vi "Temperature Controller.vi"(1 "Action":T7=enum."Identify", 2 "Parameters":variant) -> (6 "Output":variant, 7 "Stop":bool)   [LabVIEW 2024]
doc: "This VI reads a single reading from a Keithley 2001 multimeter. The stop boolean is always false. If no reading is obtained a single zero is returned.\nScott Hannahs, NHMFL-FSU, Nov 1993"
uses:
  Sub Controls/Instrument Actions.ctl
  Sub Controls/Instrument Match.ctl
  Sub Controls/Public.ctl
  Sub Controls/Factory Reset.ctl
  Sub Controls/Scan Output.ctl
  Sub Controls/Instrument IDN.ctl
  Sub Controls/User Event Command.ctl
  <vilib>/Utility/error.llb/Trim Whitespace One-Sided.vi
panel:
  in  "Factory Reset":T1
  in  "CryoCon 62 Channel":enum16{"A", "B"}(ring) caption="Channel"
  in  "LakeShore 372 Channel":T2(ring) caption="Channel"
  out "Instrument Name":string
  in  "LakeShore 370 Channel":T3(ring) caption="Channel"
  in  "LakeShore 340 Channel":enum16{"A", "B", "C", "D"}(ring) caption="Channel"
  in  "Measurement Type":T4(radio)
  out "Title":string
  in  "Public":T5
  in  "Address":u16(ring) items=["GPIB 0 - Address 8", "GPIB 0 - Address 9", "GPIB 0 - Address 11", "GPIB 0 - Address 12", "GPIB 0 - Address 13"]
  out "Model":string
  in  "Instruments":T6[](array[typedef])=[{"Model"="MODEL370", "Manufacturer"="LSCI", "Term Character"="", "Wait Time (mS)"=0, "Wait for SRQ"=FALSE, "Type"="Temperature Controller"}, {"Model"="MODEL340", "Manufacturer"="LSCI", "Term Character"="", "Wait Time (mS)"=0, "Wait for SRQ"=FALSE, "Type"="Temperature Controller"}, {"Model"="MODEL336", "Manufacturer"="LSCI", "Term Character"="", "Wait Time (mS)"=0, "Wait for SRQ"=FALSE, "Type"="Temperature Controller"}, {"Model"="Model 62", "Manufacturer"="Cryocon", "Term Character"="", "Wait Time (mS)"=0, "Wait for SRQ"=FALSE, "Type"="Temperature Controller"}, {"Model"="MODEL372", "Manufacturer"="LSCI", "Term Character"="", "Wait Time (mS)"=0, "Wait for SRQ"=FALSE, "Type"="Temperature Controller"}, {"Model"="24C", "Manufacturer"="Cryo-con", "Term Character"="", "Wait Time (mS)"=0, "Wait for SRQ"=FALSE, "Type"="Temperature Controller"}, {"Model"="Model", "Manufacturer"="Cryocon", "Term Character"="", "Wait Time (mS)"=0, "Wait for SRQ"=FALSE, "Type"="Temperature Controller"}, {"Model"="MODEL331S", "Manufacturer"="LSCI", "Term Character"="", "Wait Time (mS)"=0, "Wait for SRQ"=FALSE, "Type"="Temperature Controller"}]
  out "Measurement":dbl[](array[numeric]) format="%^_7e"
  in  "VISA resource name":refnum<visa-resource-name>
  # "Term Char"
  # "Wait Time (mS)"
  # "Wait for SRQ?"
  # "Type"
  # "Manufacturer"
  # "Model"
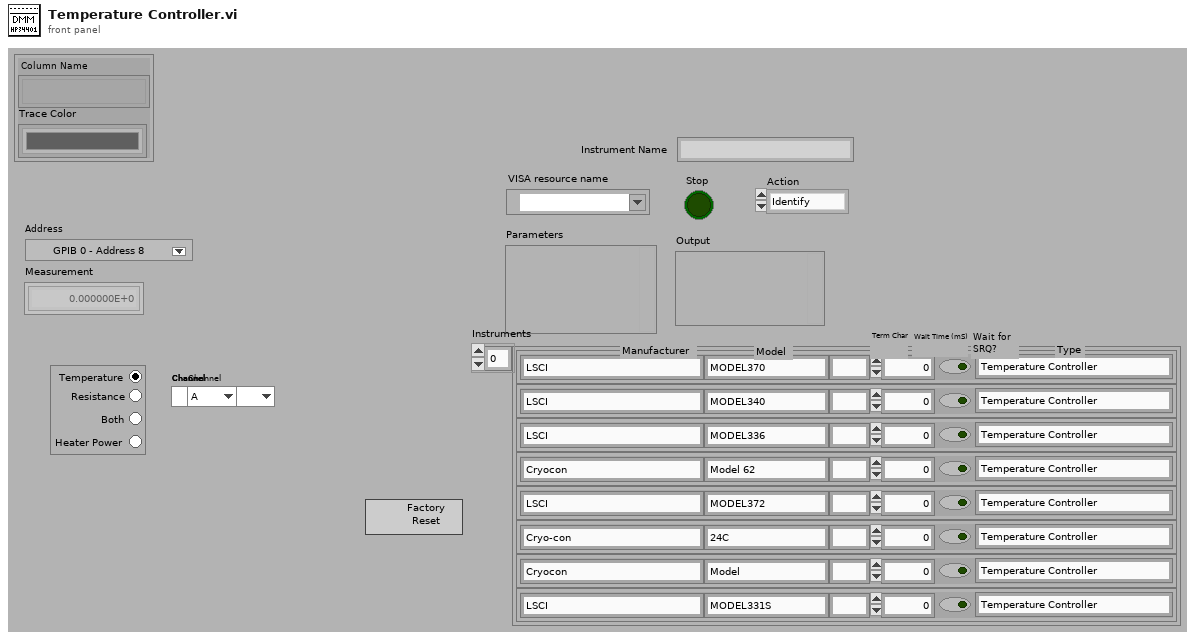
[diagram p1: front panel]
types:
  T1 = typedef "Factory Reset.ctl" = bool
  T2 = enum16{"A", "1", "2", "3", "4", "5", "6", "7", "8", "9", "10", "11", "12", "13", "14", "15", "16"}
  T3 = enum16{"1", "2", "3", "4", "5", "6", "7", "8", "9", "10", "11", "12", "13", "14", "15", "16"}
  T4 = enum32{"Temperature", "Resistance", "Both", "Heater Power"}
  T5 = typedef "Public.ctl" = cluster{"Column Name":string[], "Trace Color":u32[]}
  T6 = typedef "Instrument Match.ctl" = cluster{"Model":string, "Manufacturer":string, "Term Character":string, "Wait Time (mS)":u32, "Wait for SRQ":bool, "Type":string}
  T7 = typedef "Instrument Actions.ctl" = enum16{"Scan", "Identify", "New", "Configure", "Initialize", "Test", "Read", "Close"}
  T8 = typedef "Scan Output.ctl" = cluster{"Manufacturer":string, "Model":string, "Info":string, "Revision":string, "error out":errorcluster}
  T9 = typedef "Instrument IDN.ctl" = cluster{"VISA Address":string, "Status":u16, "Manufacturer":string, "Model":string, "Info":string, "Info 2":string, "Misc Data":variant}
  T10 = typedef "User Event Command.ctl" = enum32{"Stop Config"}
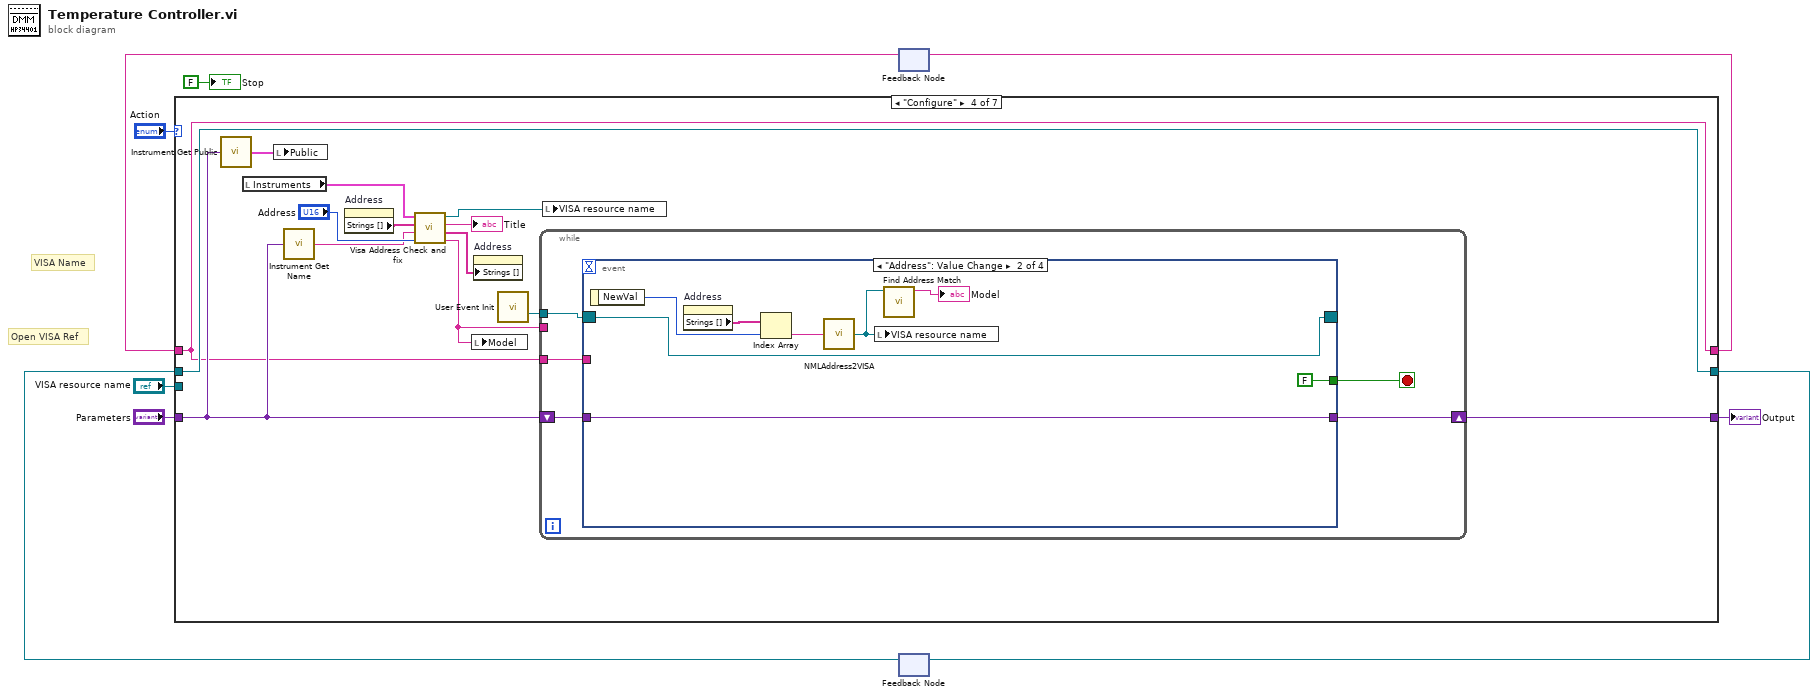
[diagram p0: block diagram]
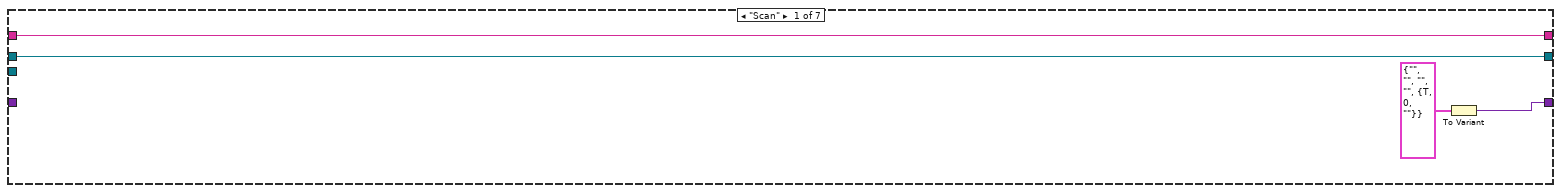
[diagram p2: hidden frame]
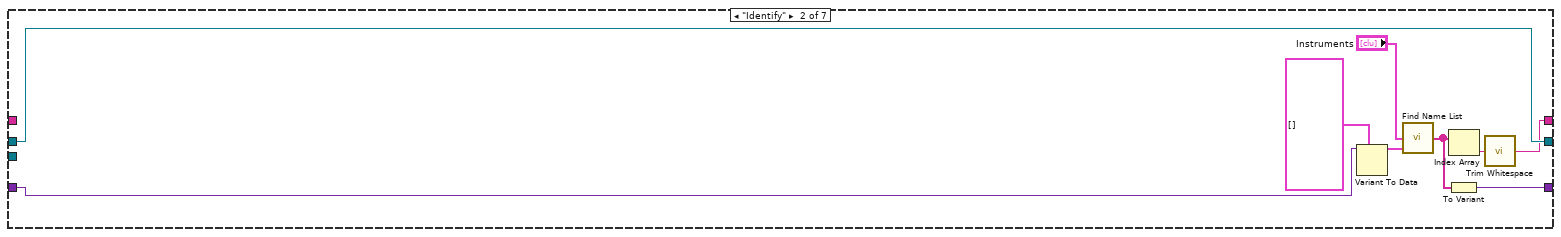
[diagram p3: hidden frame]
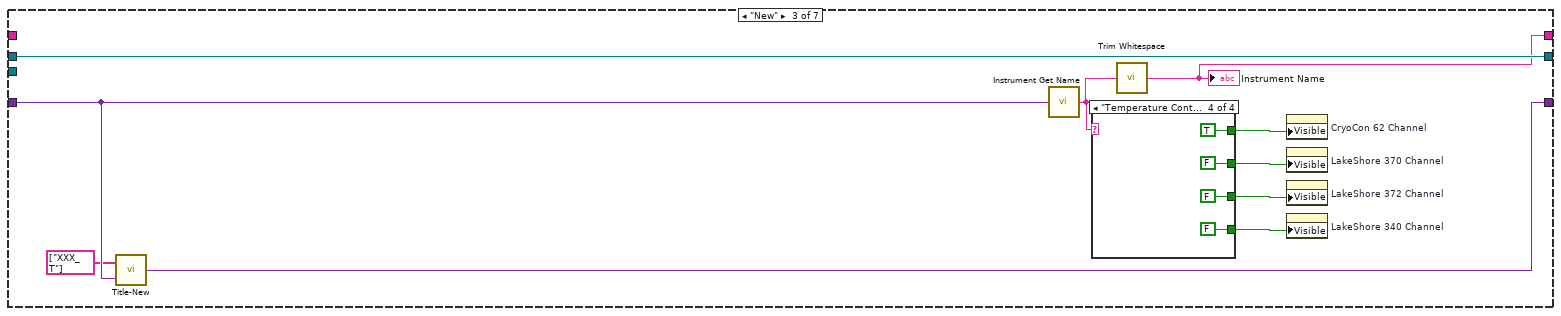
[diagram p4: hidden frame]
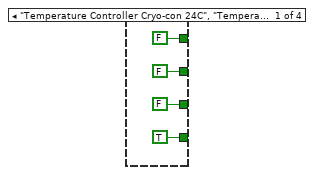
[diagram p5: hidden frame]
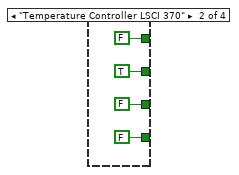
[diagram p6: hidden frame]
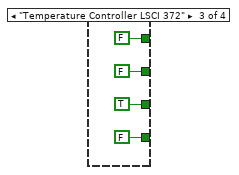
[diagram p7: hidden frame]
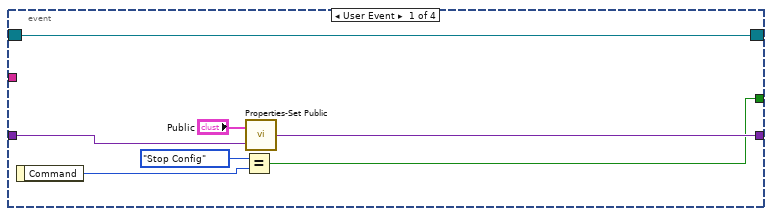
[diagram p8: hidden frame]
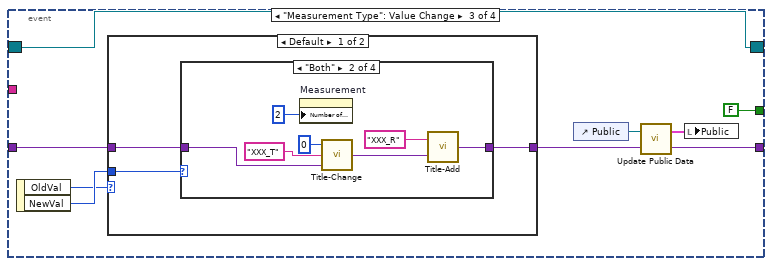
[diagram p9: hidden frame]
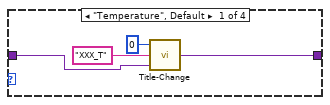
[diagram p10: hidden frame]
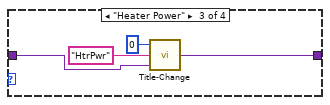
[diagram p11: hidden frame]
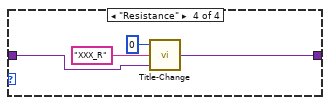
[diagram p12: hidden frame]
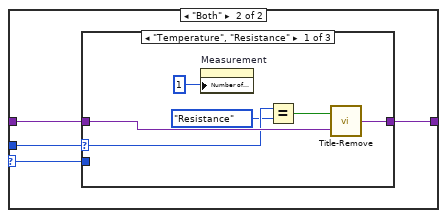
[diagram p13: hidden frame]
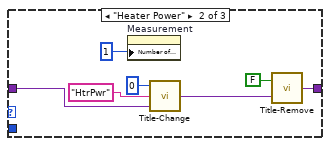
[diagram p14: hidden frame]
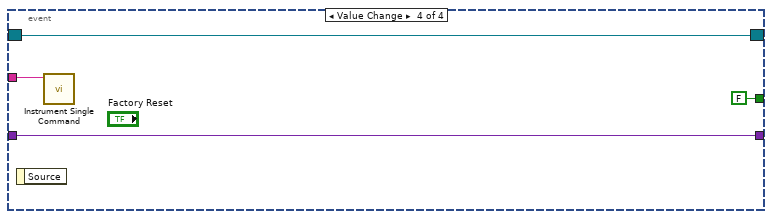
[diagram p16: hidden frame]
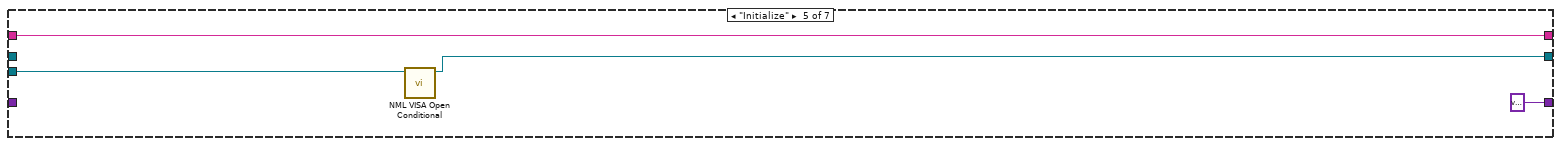
[diagram p17: hidden frame]
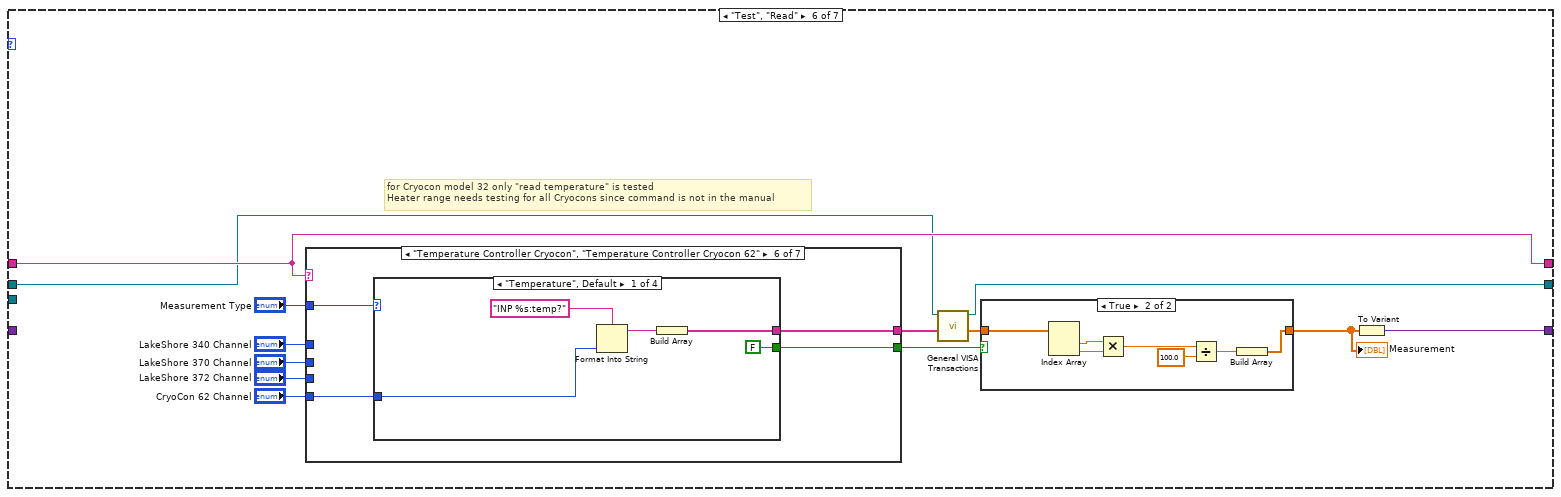
[diagram p18: hidden frame]
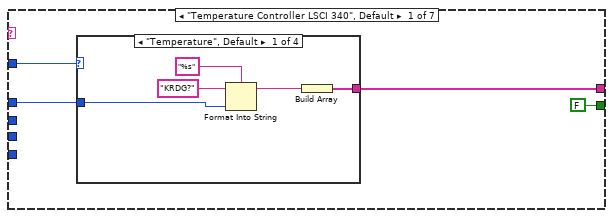
[diagram p20: hidden frame]
diagram:
  # "VISA Name"
  # "Open VISA Ref"
  n1 = feedback #1() -> (w6:string)  [unwired: 1 in]
  n2 = feedback #2() -> (w3:refnum<visa-resource-name>)  [unwired: 1 in]
  n3 = case shown="\"Configure\"" "Action" {
    tunnel: [w13 w22 w32 w57 variant ("Variant") w142 variant ("Variant")] -> w8
    tunnel: "VISA resource name" -> [_ _ _ _ w139 _ _]
    tunnel: [w12 w14 w23 w49 w137 w151 w328] -> w1
    tunnel: w6 -> [w12 _ _ w49 w137 w151 w328]
    tunnel: "Parameters" -> [_ w21 w30 w53 _ _ _]
    tunnel: [w11 w16 w31 w54 w136 w152 refnum<visa-resource-name> refnum ("Open VISA Resource name")] -> w4
    tunnel: w3 -> [w11 w16 w31 w54 _ w143 w326]
    frame "Scan" {
      n4 = To Variant(anything=T8 {"Manufacturer"="", "Model"="", "Info"="", "Revision"="", "error out"={"status"=TRUE, "code"=0, "source"=""}} ("Scan Output")) -> (Variant=w13:variant)
    }
    frame "Identify" {
      n5 = Variant To Data(type=T9[] [], Variant=w21) -> (data=w19:T9[])  [unwired: 1 in, 1 out]
      n6 = call "Find Name List.vi"("Bus Scan"=w19, "Instruments"="Instruments") -> ("Names"=w15:string[])  [unwired: 1 in]
      n7 = Index Array(array=w15) -> (element=w17:string)  [unwired: 1 in]
      n8 = To Variant(anything=w15) -> (Variant=w22:variant)
      n9 = call <vilib>:"Trim Whitespace.vi"("string"=w17) -> ("trimmed string"=w14:string)  [unwired: 1 in]
    }
    frame "New" {
      n10 = call "Title-New.vi"("Parameters"=w30, "Array"=string[] ["XXX_T"]) -> ("Instrument Prop"=w32:variant)
      n11 = call "Instrument Get Name.vi"("Parameters"=w30) -> ("Type"=w29:string)
      n12 = case shown="\"Temperature Controller Cryocon\", \"Temperature Controller Cryocon 62\", \"Temperature Controller LSCI 331S\"" w29 {
        tunnel: [TRUE ("Visible") FALSE ("Visible") FALSE ("Visible") FALSE ("Visible")] -> w28
        tunnel: [FALSE ("Visible") TRUE ("Visible") FALSE ("Visible") FALSE ("Visible")] -> w27
        tunnel: [FALSE ("Visible") FALSE ("Visible") FALSE ("Visible") TRUE ("Visible")] -> w26
        tunnel: [FALSE FALSE ("Visible") TRUE ("Visible") FALSE] -> w24
        frame "Temperature Controller Cryo-con 24C", "Temperature Controller LSCI 336 ", "Temperature Controller LSCI 340", Default {
        }
        frame "Temperature Controller LSCI 370" {
        }
        frame "Temperature Controller LSCI 372" {
        }
        frame "Temperature Controller Cryocon", "Temperature Controller Cryocon 62", "Temperature Controller LSCI 331S" {
        }
      }
      n13 = call <vilib>:"Trim Whitespace.vi"("string"=w29) -> ("trimmed string"=w23:string)  [unwired: 1 in]
      "Instrument Name" <- w23
      n14 = property on="CryoCon 62 Channel" class="Enum (strict)"("Visible"=w26) -> ()  [unwired: 2 in, 2 out]
      n15 = property on="LakeShore 370 Channel" class="Enum (strict)"("Visible"=w27) -> ()  [unwired: 2 in, 2 out]
      n16 = property on="LakeShore 372 Channel" class="Enum (strict)"("Visible"=w24) -> ()  [unwired: 2 in, 2 out]
      n17 = property on="LakeShore 340 Channel" class="Enum (strict)"("Visible"=w28) -> ()  [unwired: 2 in, 2 out]
    }
    frame "Configure" {
      n18 = call "Instrument Get Public.vi"("Variant"=w53) -> ("Public"=w58:T5)
      n19 = local read "Instruments"() -> (w60:T6[])
      n20 = local write "Public"(w58) -> ()
      n21 = call "Instrument Get Name.vi"("Parameters"=w53) -> ("Type"=w52:string)
      n22 = property on="Address" class="Ring (strict)"() -> ("Strings []"=w61:string[])  [unwired: 2 in, 2 out]
      n23 = call "Visa Address Check and fix.vi"("Address"="Address", "Name"=w52, "NML Addresses"=w61, "Instruments"=w60) -> ("Model"=w59:string, "NML Addresses"=w50:string[], "Title"=→"Title":string, "VISA resource name"=w55:refnum<visa-resource-name>)  [unwired: 2 out]
      n24 = local write "Model"(w59) -> ()
      n25 = property on="Address" class="Ring (strict)"("Strings []"=w50) -> ()  [unwired: 2 in, 2 out]
      n26 = call "User Event Init.vi"() -> ("Event Registration Refnum"=w56:refnum<event-registration>)  [unwired: 14 in, 1 out]
      n27 = while {
        tunnel: w59 -> [_]
        tunnel: w56 -> [w64]
        shift-right: [w67] -> w57
        shift-left: w53 -> [w65]
        tunnel: w49 -> [w63]
        stop <- w66 stop-if-true
        n28 = event shown="[1] \"Address\": Value Change" {
          selector: w64 -> [w68 w76 w90 w132]
          dyn-events: [w68 w76 w90 w132] -> _
          timeout: _ -> [_ _ _ _]
          tunnel: [w72 w77 w91 w134] -> w67
          tunnel: [w70 FALSE FALSE FALSE] -> w66
          tunnel: w65 -> [w73 w77 w88 w134]
          tunnel: w63 -> [_ _ _ w135]
          event User Event {
            n29 = event-data() -> ("Command"=w74:T10)  [unwired: 1 in]
            n30 = Equal?(x=User_Event_Command."Stop Config", y=w74) -> (x = y?=w70:bool)
            n31 = call "Properties-Set Public.vi"("Variant"=w73, "New Public"="Public") -> ("Variant 2"=w72:variant)
          }
          event "Address": Value Change {
            n32 = event-data() -> ("NewVal"=w82:u16)  [unwired: 1 in]
            n33 = property on="Address" class="Ring (strict)"() -> ("Strings []"=w79:string[])  [unwired: 2 in, 2 out]
            n34 = Index Array(array=w79, index=w82) -> (element=w80:string)
            n35 = call "NMLAddress2VISA.vi"("NML Address"=w80) -> ("VISA resource name"=w75:refnum<visa-resource-name>)
            n36 = local write "VISA resource name"(w75) -> ()
            n37 = call "Find Address Match.vi"("VISA resource name"=w75) -> ("Model"=→"Model":string)  [unwired: 3 in, 3 out]
          }
          event "Measurement Type": Value Change {
            n38 = event-data() -> ("OldVal"=w86:T4, "NewVal"=w87:T4)  [unwired: 1 in]
            n39 = case shown="Default" w86 {
              selector: w86 -> [_ w114]
              tunnel: [w92 w117] -> w89
              tunnel: w88 -> [w93 w116]
              tunnel: w87 -> [w94 w115]
              frame Default {
                n40 = case shown="\"Both\"" w94 {
                  tunnel: w93 -> [w96 w101 w107 w111]
                  tunnel: [w95 w104 w106 w110] -> w92
                  frame "Temperature", Default {
                    n41 = call "Title-Change.vi"("Parameters"=w96, "New Title"="XXX_T" ("Title"), "Index"=0) -> ("Variant"=w95:variant)
                  }
                  frame "Both" {
                    n42 = property on="Measurement" class="Arr (strict)"("Number of Columns"=u32 2) -> ()  [unwired: 2 in, 2 out]
                    n43 = call "Title-Change.vi"("Parameters"=w101, "New Title"="XXX_T" ("Title"), "Index"=0) -> ("Variant"=w100:variant)
                    n44 = call "Title-Add.vi"("Parameters"=w100, "String"="XXX_R") -> ("Variant"=w104:variant)
                  }
                  frame "Heater Power" {
                    n45 = call "Title-Change.vi"("Parameters"=w107, "New Title"="HtrPwr" ("Title"), "Index"=0) -> ("Variant"=w106:variant)
                  }
                  frame "Resistance" {
                    n46 = call "Title-Change.vi"("Parameters"=w111, "New Title"="XXX_R" ("Title"), "Index"=0) -> ("Variant"=w110:variant)
                  }
                }
              }
              frame "Both" {
                n47 = case shown="\"Temperature\", \"Resistance\"" w115 {
                  selector: w115 -> [w121 _ _]
                  tunnel: w116 -> [w123 w126 w131]
                  tunnel: [w122 w130 w131] -> w117
                  tunnel: w114 -> [_ _ _]
                  frame "Temperature", "Resistance" {
                    n48 = property on="Measurement" class="Arr (strict)"("Number of Columns"=u32 1) -> ()  [unwired: 2 in, 2 out]
                    n49 = Equal?(x=w121, y=T4."Resistance") -> (x = y?=w119:bool)
                    n50 = call "Title-Remove.vi"("Parameters"=w123, "Remove First"=w119) -> ("Variant"=w122:variant)
                  }
                  frame "Heater Power" {
                    n51 = property on="Measurement" class="Arr (strict)"("Number of Columns"=u32 1) -> ()  [unwired: 2 in, 2 out]
                    n52 = call "Title-Change.vi"("Parameters"=w126, "New Title"="HtrPwr" ("Title"), "Index"=0) -> ("Variant"=w127:variant)
                    n53 = call "Title-Remove.vi"("Parameters"=w127, "Remove First"=FALSE) -> ("Variant"=w130:variant)
                  }
                  frame "Both" {
                  }
                }
              }
            }
            n54 = control-ref of="Public"() -> (w84:refnum<vi>)
            n55 = call "Update Public Data.vi"("Variant In"=w89, "Public 2"=w84) -> ("Variant Out"=w91:variant, "Public"=w83:T5)
            n56 = local write "Public"(w83) -> ()
          }
          event Value Change {
            n57 = event-data() -> ()  [unwired: 1 in, 1 out]
            n58 = call "Instrument Single Command.vi"("VISA Name"=w135) -> ()  [unwired: 10 in, 1 out]
          }
        }
      }
      n59 = local write "VISA resource name"(w55) -> ()
    }
    frame "Initialize" {
      n60 = call "NML VISA Open Conditional.vi"("VISA resource name"=w139) -> ("dup VISA Session"=w136:refnum<visa-resource-name>)  [unwired: 8 in, 2 out]
    }
    frame "Test", "Read" {
      # "for Cryocon model 32 only \"read temperature\" is tested\nHeater range needs testing for all Cryocons since command is not in the manual"
      n61 = case shown="\"Temperature Controller Cryocon\", \"Temperature Controller Cryocon 62\"" w151 {
        tunnel: [w162 w185 w209 w231 w255 w279 w304] -> w149
        tunnel: "Measurement Type" -> [w164 w187 w210 w233 w256 w278 w303]
        tunnel: "LakeShore 340 Channel" -> [w163 w186 _ _ _ _ w301]
        tunnel: "LakeShore 370 Channel" -> [_ _ _ w232 _ _ _]
        tunnel: "CryoCon 62 Channel" -> [_ _ w207 _ _ w277 _]
        tunnel: [FALSE FALSE FALSE FALSE FALSE w276 w302] -> w145
        tunnel: "LakeShore 372 Channel" -> [_ _ _ _ w253 _ _]
        frame "Temperature Controller LSCI 340", Default {
          n62 = case shown="\"Temperature\", Default" w164 {
            tunnel: [w169 w174 w181 w182] -> w162
            tunnel: w163 -> [w167 w170 w180 _]
            frame "Temperature", Default {
              n63 = Format Into String(format string="%s", initial string="KRDG?" ("Format String"), w167) -> (resulting string=w165:string)  [unwired: 1 in, 1 out]
              n64 = Build Array(w165) -> (w169:string[])
            }
            frame "Resistance" {
              n65 = Format Into String(format string="%s", initial string="SRDG?" ("Format String"), w170) -> (resulting string=w172:string)  [unwired: 1 in, 1 out]
              n66 = Build Array(w172) -> (w174:string[])
            }
            frame "Both" {
              w179 = "%s" ("format string")
              n67 = Format Into String(format string=w179, initial string="KRDG?" ("Format String"), w180) -> (resulting string=w178:string)  [unwired: 1 in, 1 out]
              n68 = Format Into String(format string=w179, initial string="SRDG?" ("Format String"), w180) -> (resulting string=w175:string)  [unwired: 1 in, 1 out]
              n69 = Build Array(w178, w175) -> (w181:string[])
            }
            frame "Heater Power" {
              n70 = Build Array("HTR?" ("Format String")) -> (w182:string[])
            }
          }
        }
        frame "Temperature Controller LSCI 336" {
          n71 = case shown="\"Both\"" w187 {
            tunnel: [w192 w197 w204 w205] -> w185
            tunnel: w186 -> [w190 w193 w203 _]
            frame "Temperature", Default {
              n72 = Format Into String(format string="%s", initial string="KRDG? " ("Format String"), w190) -> (resulting string=w188:string)  [unwired: 1 in, 1 out]
              n73 = Build Array(w188) -> (w192:string[])
            }
            frame "Resistance" {
              n74 = Format Into String(format string="%s", initial string="SRDG? " ("Format String"), w193) -> (resulting string=w195:string)  [unwired: 1 in, 1 out]
              n75 = Build Array(w195) -> (w197:string[])
            }
            frame "Both" {
              w202 = "%s" ("format string")
              n76 = Format Into String(format string=w202, initial string="KRDG? " ("Format String"), w203) -> (resulting string=w201:string)  [unwired: 1 in, 1 out]
              n77 = Format Into String(format string=w202, initial string="SRDG? " ("Format String"), w203) -> (resulting string=w198:string)  [unwired: 1 in, 1 out]
              n78 = Build Array(w201, w198) -> (w204:string[])
            }
            frame "Heater Power" {
              n79 = Build Array("HTR? 1" ("Format String")) -> (w205:string[])
            }
          }
        }
        frame "Temperature Controller LSCI 331S" {
          n80 = case shown="\"Both\"" w210 {
            tunnel: [w215 w220 w227 w228] -> w209
            tunnel: w207 -> [w213 w216 w226 _]
            frame "Temperature", Default {
              n81 = Format Into String(format string="%s", initial string="KRDG? " ("Format String"), w213) -> (resulting string=w211:string)  [unwired: 1 in, 1 out]
              n82 = Build Array(w211) -> (w215:string[])
            }
            frame "Resistance" {
              n83 = Format Into String(format string="%s", initial string="SRDG? " ("Format String"), w216) -> (resulting string=w218:string)  [unwired: 1 in, 1 out]
              n84 = Build Array(w218) -> (w220:string[])
            }
            frame "Both" {
              w225 = "%s" ("format string")
              n85 = Format Into String(format string=w225, initial string="KRDG? " ("Format String"), w226) -> (resulting string=w224:string)  [unwired: 1 in, 1 out]
              n86 = Format Into String(format string=w225, initial string="SRDG? " ("Format String"), w226) -> (resulting string=w221:string)  [unwired: 1 in, 1 out]
              n87 = Build Array(w224, w221) -> (w227:string[])
            }
            frame "Heater Power" {
              n88 = Build Array("HTR? 1" ("Format String")) -> (w228:string[])
            }
          }
        }
        frame "Temperature Controller LSCI 370" {
          n89 = case shown="\"Temperature\", Default" w233 {
            tunnel: [w238 w243 w250 w251] -> w231
            tunnel: w232 -> [w236 w239 w249 _]
            frame "Temperature", Default {
              n90 = Format Into String(format string="%s", initial string="RDGK?" ("Format String"), w236) -> (resulting string=w234:string)  [unwired: 1 in, 1 out]
              n91 = Build Array(w234) -> (w238:string[])
            }
            frame "Resistance" {
              n92 = Format Into String(format string="%s", initial string="RDGR?" ("Format String"), w239) -> (resulting string=w241:string)  [unwired: 1 in, 1 out]
              n93 = Build Array(w241) -> (w243:string[])
            }
            frame "Both" {
              w248 = "%s" ("format string")
              n94 = Format Into String(format string=w248, initial string="RDGK?" ("Format String"), w249) -> (resulting string=w247:string)  [unwired: 1 in, 1 out]
              n95 = Format Into String(format string=w248, initial string="RDGR?" ("Format String"), w249) -> (resulting string=w244:string)  [unwired: 1 in, 1 out]
              n96 = Build Array(w247, w244) -> (w250:string[])
            }
            frame "Heater Power" {
              n97 = Build Array("HTR?" ("Format String")) -> (w251:string[])
            }
          }
        }
        frame "Temperature Controller LSCI 372" {
          n98 = case shown="\"Both\"" w256 {
            tunnel: [w261 w266 w273 w274] -> w255
            tunnel: w253 -> [w259 w262 w272 _]
            frame "Temperature", Default {
              n99 = Format Into String(format string="%s", initial string="RDGK?" ("Format String"), w259) -> (resulting string=w257:string)  [unwired: 1 in, 1 out]
              n100 = Build Array(w257) -> (w261:string[])
            }
            frame "Resistance" {
              n101 = Format Into String(format string="%s", initial string="RDGR?" ("Format String"), w262) -> (resulting string=w264:string)  [unwired: 1 in, 1 out]
              n102 = Build Array(w264) -> (w266:string[])
            }
            frame "Both" {
              w271 = "%s" ("format string")
              n103 = Format Into String(format string=w271, initial string="RDGK?" ("Format String"), w272) -> (resulting string=w270:string)  [unwired: 1 in, 1 out]
              n104 = Format Into String(format string=w271, initial string="RDGR?" ("Format String"), w272) -> (resulting string=w267:string)  [unwired: 1 in, 1 out]
              n105 = Build Array(w270, w267) -> (w273:string[])
            }
            frame "Heater Power" {
              n106 = Build Array("HTR?" ("Format String")) -> (w274:string[])
            }
          }
        }
        frame "Temperature Controller Cryocon", "Temperature Controller Cryocon 62" {
          n107 = case shown="\"Temperature\", Default" w278 {
            tunnel: [w284 w289 w296 w299] -> w279
            tunnel: w277 -> [w281 w286 w291 _]
            tunnel: [FALSE FALSE FALSE TRUE] -> w276
            frame "Temperature", Default {
              n108 = Format Into String(format string="INP %s:temp?" ("Format String"), w281) -> (resulting string=w283:string)  [unwired: 2 in, 1 out]
              n109 = Build Array(w283) -> (w284:string[])
            }
            frame "Resistance" {
              n110 = Format Into String(format string="INP %s:senpr?" ("Format String"), w286) -> (resulting string=w288:string)  [unwired: 2 in, 1 out]
              n111 = Build Array(w288) -> (w289:string[])
            }
            frame "Both" {
              n112 = Format Into String(format string="INP %s:temp?" ("Format String"), w291) -> (resulting string=w295:string)  [unwired: 2 in, 1 out]
              n113 = Format Into String(format string="INP %s:senpr?" ("Format String"), w291) -> (resulting string=w290:string)  [unwired: 2 in, 1 out]
              n114 = Build Array(w295, w290) -> (w296:string[])
            }
            frame "Heater Power" {
              n115 = Build Array("Heat:htrr?" ("Format String"), "Heat:rang?" ("element")) -> (w299:string[])
            }
          }
        }
        frame "Temperature Controller Cryo-con 24C" {
          n116 = case shown="\"Heater Power\"" w303 {
            tunnel: [w309 w314 w321 w324] -> w304
            tunnel: w301 -> [w306 w311 w316 _]
            tunnel: [FALSE FALSE FALSE TRUE] -> w302
            frame "Temperature", Default {
              n117 = Format Into String(format string="INP %s:temp?" ("Format String"), w306) -> (resulting string=w308:string)  [unwired: 2 in, 1 out]
              n118 = Build Array(w308) -> (w309:string[])
            }
            frame "Resistance" {
              n119 = Format Into String(format string="INP %s:senpr?" ("Format String"), w311) -> (resulting string=w313:string)  [unwired: 2 in, 1 out]
              n120 = Build Array(w313) -> (w314:string[])
            }
            frame "Both" {
              n121 = Format Into String(format string="INP %s:senpr?" ("Format String"), w316) -> (resulting string=w320:string)  [unwired: 2 in, 1 out]
              n122 = Format Into String(format string="INP %s:temp?" ("Format String"), w316) -> (resulting string=w315:string)  [unwired: 2 in, 1 out]
              n123 = Build Array(w320, w315) -> (w321:string[])
            }
            frame "Heater Power" {
              n124 = Build Array("Loop 1:htrr?" ("Format String"), "Loop 1:rang?" ("element")) -> (w324:string[])
            }
          }
        }
      }
      n125 = call "General VISA Transactions.vi"("Array"=w149, "Open VISA Resource name"=w143) -> ("Measurement"=w144:dbl[], "dup VISA session"=w152:refnum<visa-resource-name>)  [unwired: 2 in, 2 out]
      n126 = case shown="True" w145 {
        tunnel: w144 -> [w153 w160]
        tunnel: [w153 w154] -> w141
        frame False {
        }
        frame True {
          n127 = Index Array(array=w160) -> (element #1=w158:dbl, element #2=w159:dbl)  [unwired: 2 in]
          n128 = Multiply(x=w158, y=w159) -> (x*y=w157:dbl)
          n129 = Divide(x=w157, y=100.0) -> (x/y=w155:dbl)
          n130 = Build Array(w155) -> (w154:dbl[])
        }
      }
      "Measurement" <- w141
      n131 = To Variant(anything=w141) -> (Variant=w142:variant)
    }
    frame "Close" {
      n132 = call "NML VISA Close.vi"("VISA resource name"=w326) -> ()  [unwired: 10 in, 1 out]
    }
  }
  "Output" <- w8
  n133 = feedback-in #1(w1) -> ()
  n134 = feedback-in #2(w4) -> ()
  "Stop" <- FALSE ("Stop")
